vi "flow_loop_data_record.vi"() -> ()   [LabVIEW 2020]
panel:
  in  "Test Number":string
  in  "Choose Folder for Data":path
  in  "Data Collect":bool
  in  "stop (F)":bool
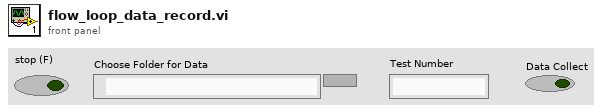
[diagram p1: front panel]
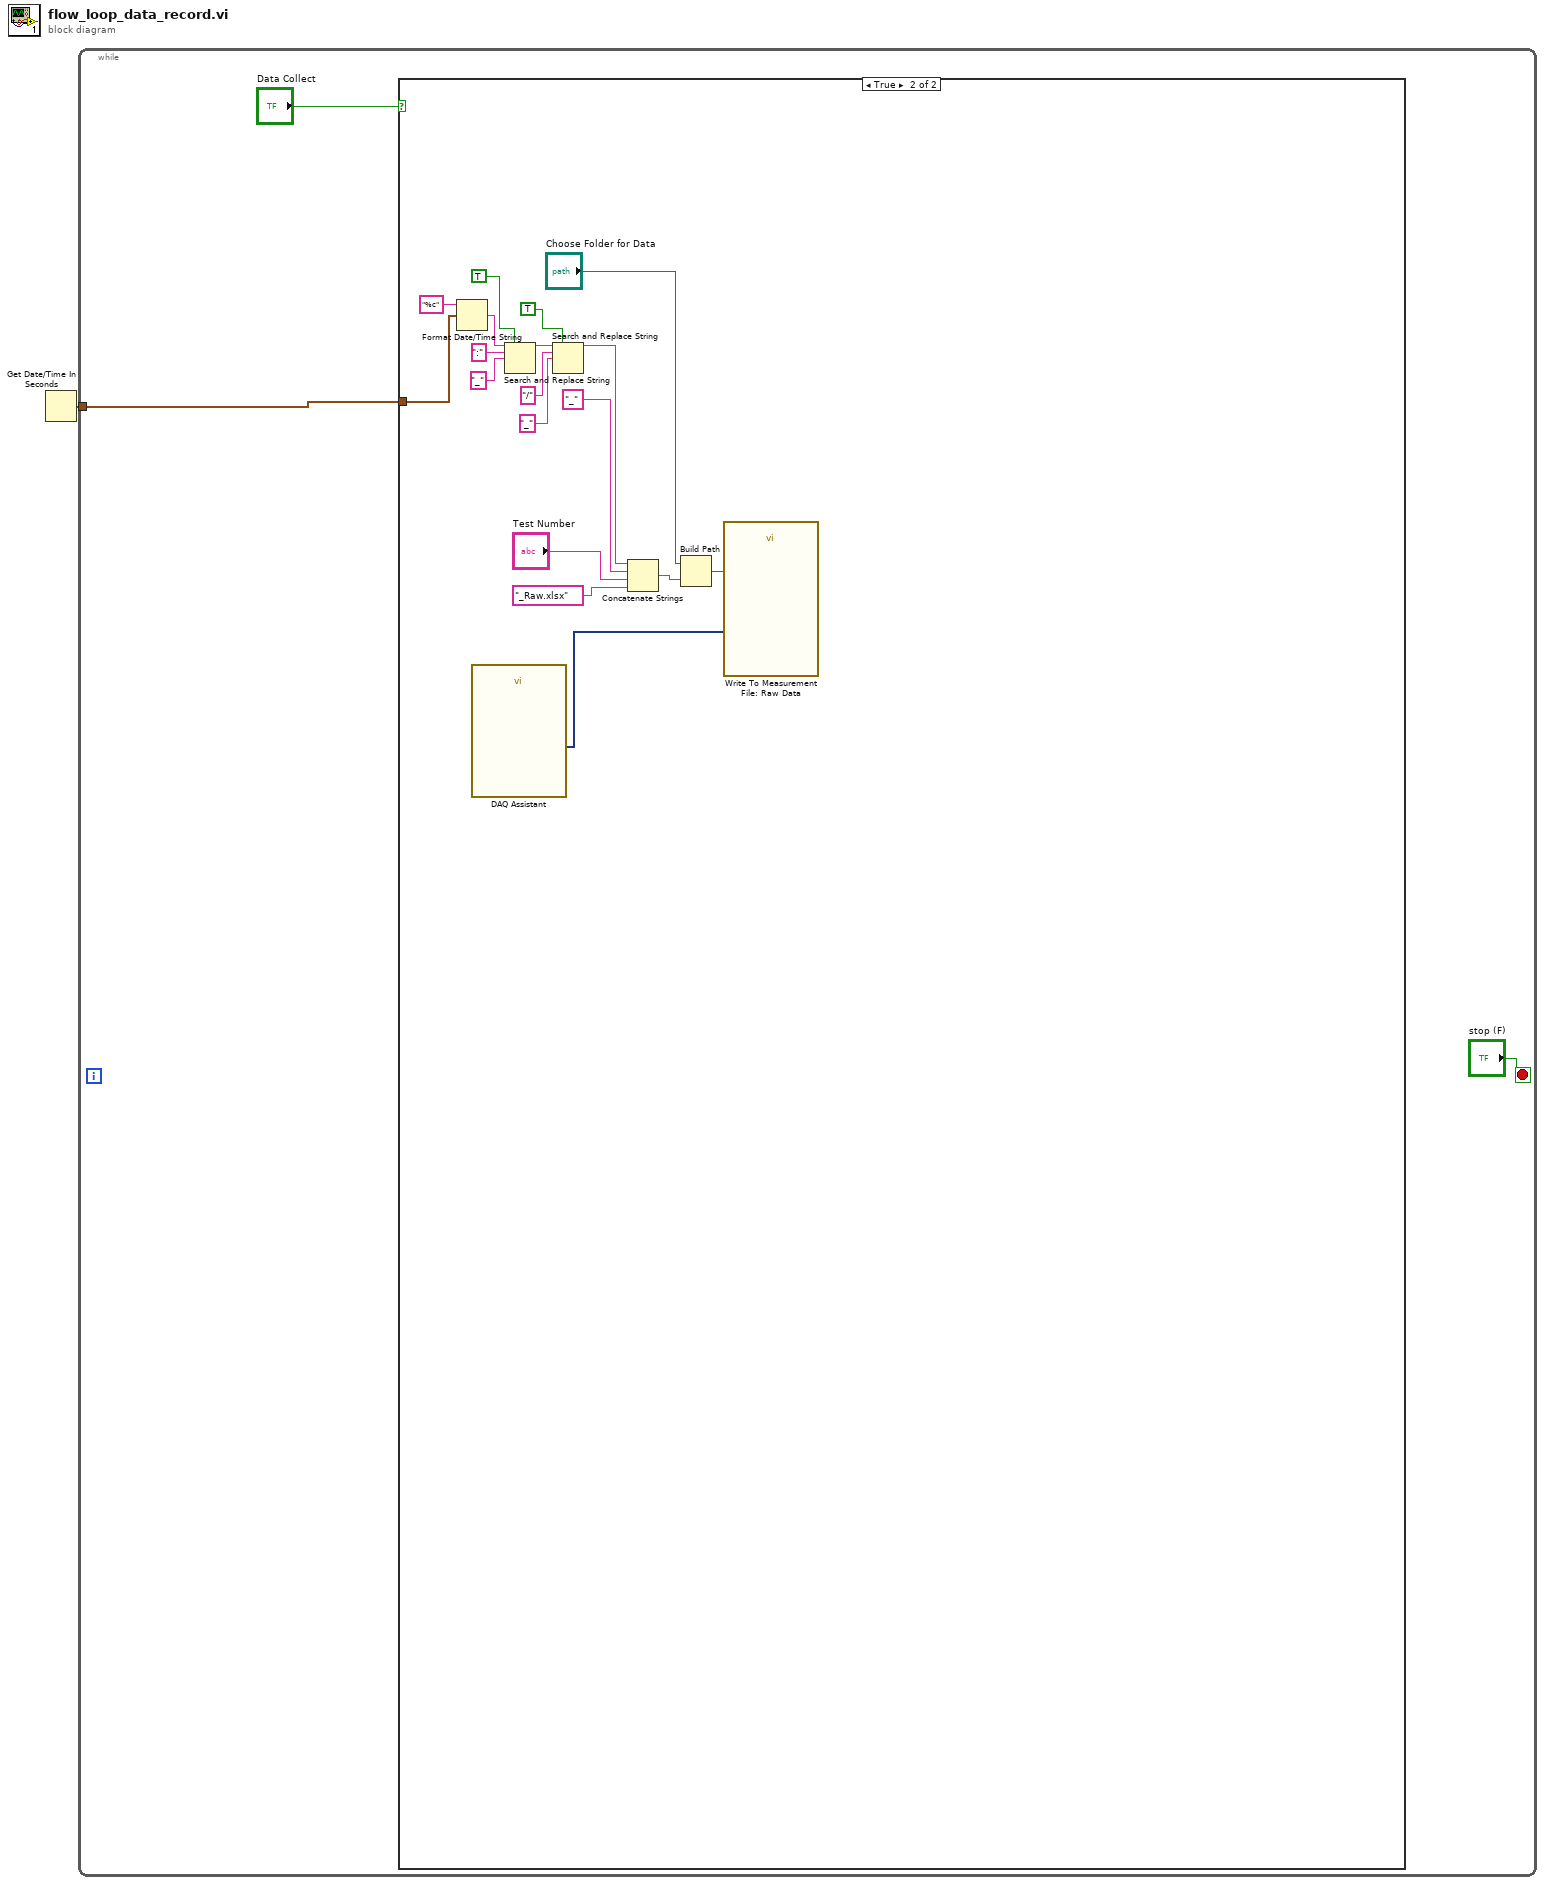
[diagram p0: block diagram]
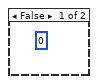
[diagram p2: hidden frame]
diagram:
  n1 = Get Date/Time In Seconds() -> (seconds since 1Jan1904=w1:timestamp)
  n2 = while {
    tunnel: w1 -> [w2]
    stop <- "stop (F)" stop-if-true
    n3 = case shown="True" "Data Collect" {
      tunnel: w2 -> [_ w9]
      frame False {
        (unwired) 0
      }
      frame True {
        n4 = Format Date/Time String(time format string (%c)="%c", seconds (now)=w9) -> (date/time string=w18:string)  [unwired: 1 in]
        n5 = call "DAQ Assistant"() -> ("data"=w6:dynamicdata)  [unwired: 16 in, 3 out]
        n6 = Search and Replace String(replace all?=TRUE ("replace all? (F)"), input string=w18, search string=":", replace string="_") -> (result string=w14:string)  [unwired: 4 in, 3 out]
        n7 = Search and Replace String(replace all?=TRUE ("replace all? (F)"), input string=w14, search string="/", replace string="_" ("replace string (\"\")")) -> (result string=w13:string)  [unwired: 4 in, 3 out]
        n8 = Concatenate Strings(w13, "_", "Test Number", "_Raw.xlsx") -> (w21:string)
        n9 = Build Path(base path="Choose Folder for Data", name or relative path=w21) -> (appended path=w20:path)
        n10 = call "Write To Measurement File: Raw Data"("Signals"=w6, "Filename"=w20) -> ()  [unwired: 15 in, 3 out]
      }
    }
  }
